vi "deleteModel.vi"(8 "Error In":errorcluster, 11 "UI Elements Cluster":T1) -> (0 "Error Out":errorcluster)   [LabVIEW 2018]
uses:
  UI Module/src/controls/mainAppElementsCluster.ctl
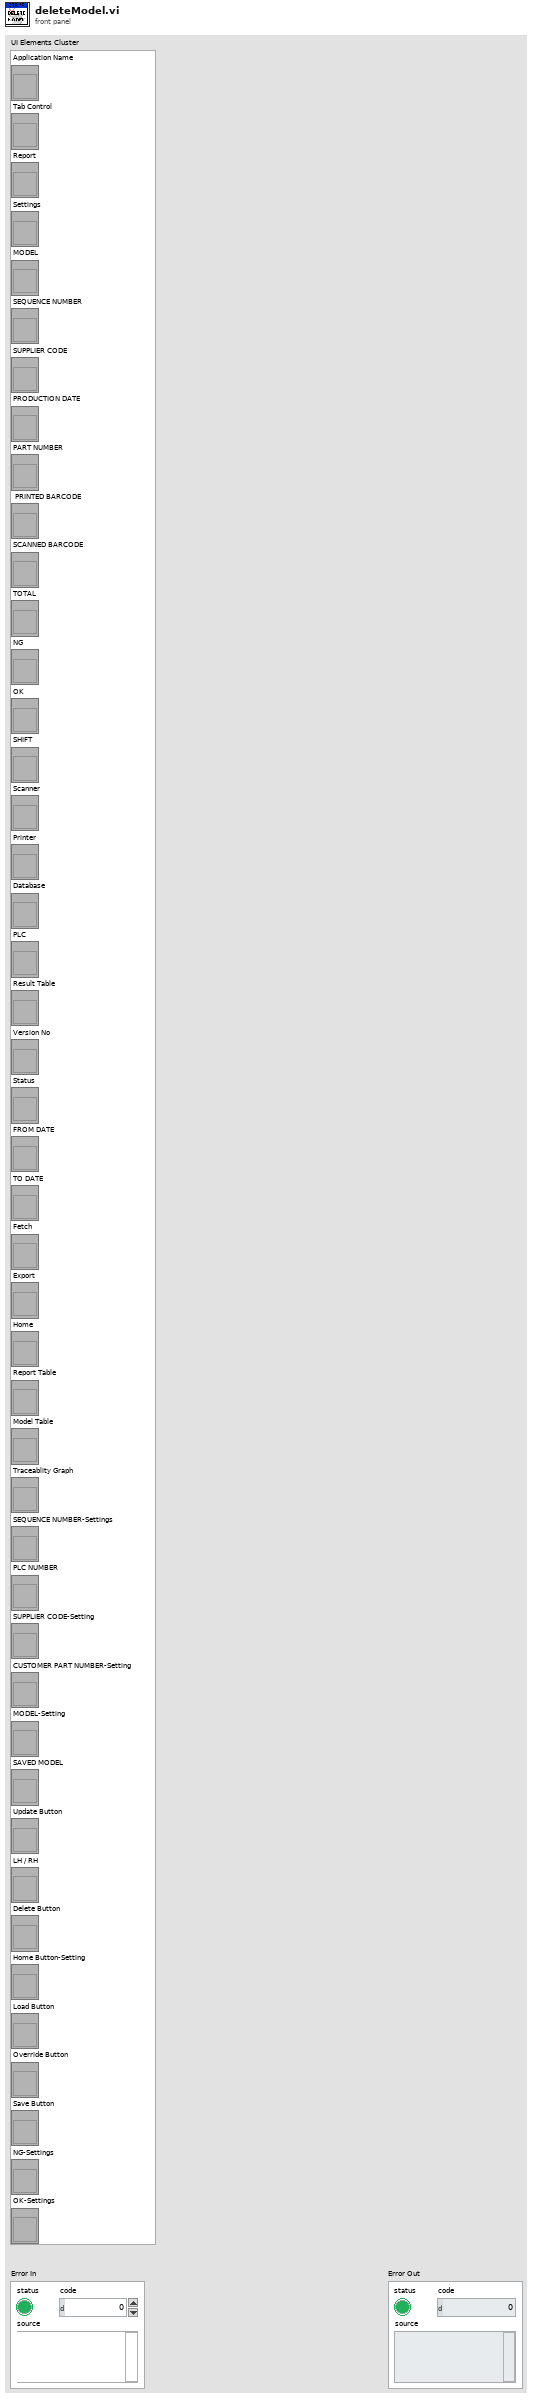
[diagram p1: front panel]
types:
  T1 = typedef "mainAppElementsCluster.ctl" = cluster{"Application Name":refnum<vi>, "Tab Control":refnum<vi>, "Status":refnum<vi>, "Version No":refnum<vi>, "Result Table":refnum<vi>, "PLC":refnum<vi>, "Database":refnum<vi>, "Printer":refnum<vi>, "Scanner":refnum<vi>, "SHIFT":refnum<vi>, "OK":refnum<vi>, "NG":refnum<vi>, "TOTAL":refnum<vi>, "SCANNED BARCODE":refnum<vi>, " PRINTED BARCODE":refnum<vi>, "PART NUMBER":refnum<vi>, "PRODUCTION DATE":refnum<vi>, "SUPPLIER CODE":refnum<vi>, "SEQUENCE NUMBER":refnum<vi>, "MODEL":refnum<vi>, "Settings":refnum<vi>, "Report":refnum<vi>, "Report Table":refnum<vi>, "Home":refnum<vi>, "Export":refnum<vi>, "Fetch":refnum<vi>, "TO DATE":refnum<vi>, "FROM DATE":refnum<vi>, "Model Table":refnum<vi>, "Traceablity Graph":refnum<vi>, "Override Button":refnum<vi>, "Load Button":refnum<vi>, "Home Button-Setting":refnum<vi>, "Delete Button":refnum<vi>, "Update Button":refnum<vi>, "Save Button":refnum<vi>, "SEQUENCE NUMBER-Settings":refnum<vi>, "PLC NUMBER":refnum<vi>, "LH / RH":refnum<vi>, "SUPPLIER CODE-Setting":refnum<vi>, "CUSTOMER PART NUMBER-Setting":refnum<vi>, "MODEL-Setting":refnum<vi>, "SAVED MODEL":refnum<vi>, "NG-Settings":refnum<vi>, "OK-Settings":refnum<vi>}
  T2 = cluster{"[0]":string, "[1]":string, "[2]":string, "[3]":string, "[4]":string, "[5]":string, "[6]":string, "[7]":string, "[8]":string}
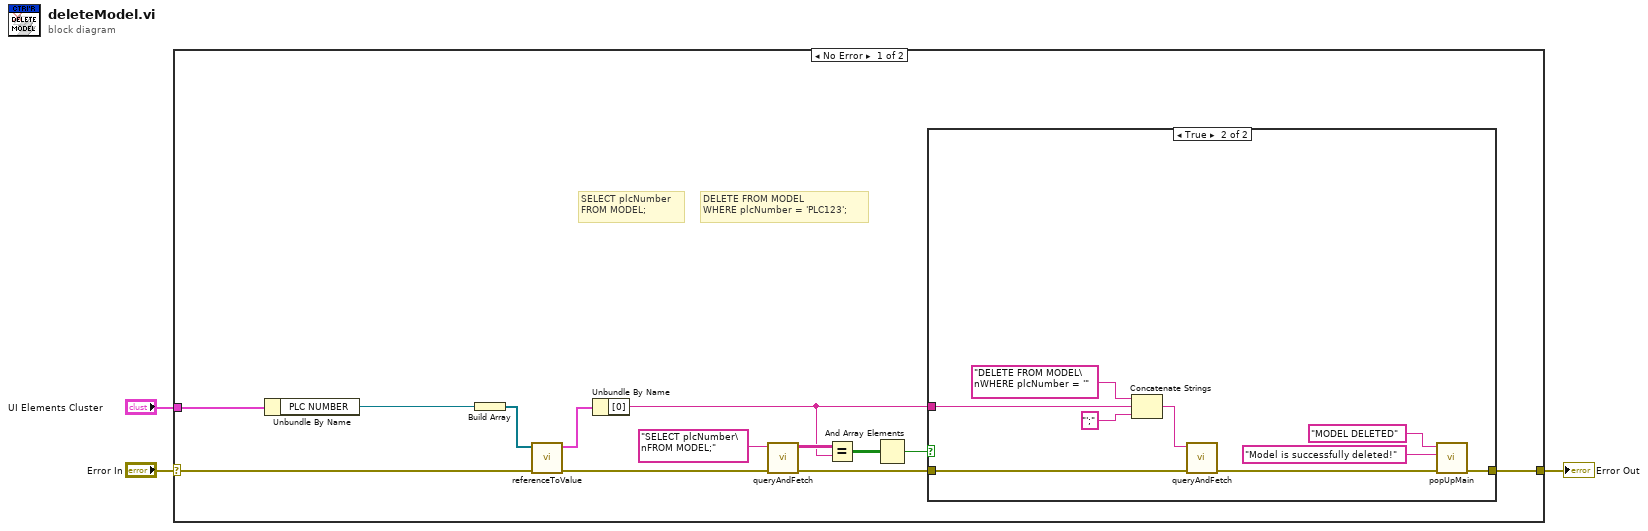
[diagram p0: block diagram]
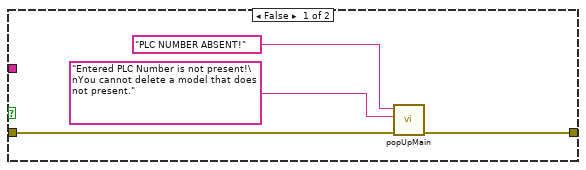
[diagram p2: hidden frame]
diagram:
  n1 = case shown="No Error" "Error In" {
    selector: "Error In" -> [w12 w30]
    tunnel: [w6 w30] -> w2
    tunnel: "UI Elements Cluster" -> [w16 _]
    frame No Error {
      # "DELETE FROM MODEL\nWHERE plcNumber = 'PLC123';"
      # "SELECT plcNumber\nFROM MODEL;"
      n2 = Unbundle By Name(w16) -> ("PLC NUMBER"=w15:refnum<vi>)
      n3 = Build Array(w15) -> (w14:refnum<vi>[])
      n4 = call "referenceToValue.vi"("Error In"=w12, "Reference Array"=w14) -> ("Error Out"=w11:errorcluster, "Value Out Cluster"=w13:T2)  [unwired: 8 in]
      n5 = Unbundle By Name(w13) -> ("[0]"=w4:string)
      n6 = call "queryAndFetch.vi"("Error In"=w11, "Query"="SELECT plcNumber\nFROM MODEL;") -> ("Error Out"=w7:errorcluster, "Result Table"=w9:string[][])  [unwired: 8 in]
      n7 = Equal?(x=w9, y=w4) -> (x = y?=w8:bool[][])
      n8 = And Array Elements(Boolean array=w8) -> (logical AND=w5:bool)
      n9 = case shown="True" w5 {
        tunnel: w7 -> [w20 w29]
        tunnel: [w19 w21] -> w6
        tunnel: w4 -> [_ w26]
        frame False {
          n10 = call "popUpMain.vi"("Error In"=w20, "Message Description"="Entered PLC Number is not present!\nYou cannot delete a model that does not present." ("Error Info"), "Message Titlt"="PLC NUMBER ABSENT!" ("Error Name")) -> ("Error Out"=w19:errorcluster)  [unwired: 7 in, 1 out]
        }
        frame True {
          n11 = Concatenate Strings("DELETE FROM MODEL\nWHERE plcNumber = '", w26, "';" ("string")) -> (w28:string)
          n12 = call "queryAndFetch.vi"("Error In"=w29, "Query"=w28) -> ("Error Out"=w22:errorcluster)  [unwired: 8 in, 1 out]
          n13 = call "popUpMain.vi"("Error In"=w22, "Message Description"="Model is successfully deleted!" ("Error Info"), "Message Titlt"="MODEL DELETED" ("Error Name")) -> ("Error Out"=w21:errorcluster)  [unwired: 7 in, 1 out]
        }
      }
    }
    frame Error {
    }
  }
  "Error Out" <- w2
